vi "AOL Z Cal-Cancel handler.vi"() -> (3 "Stop?":bool)   [LabVIEW 2020]
uses:
  Globals/gl_Calibration globals.vi
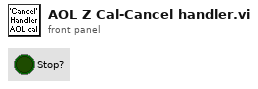
[diagram p1: front panel]
types:
  T1 = typedef "AOL Z cal process refs.ctl" = cluster{"This VI":refnum<vi>, "Abort (ind)":refnum<vi>, "Next (ind)":refnum<vi>, "Cancel":refnum<vi>, "Next":refnum<vi>, "Message":refnum<vi>, "Progress":refnum<vi>}
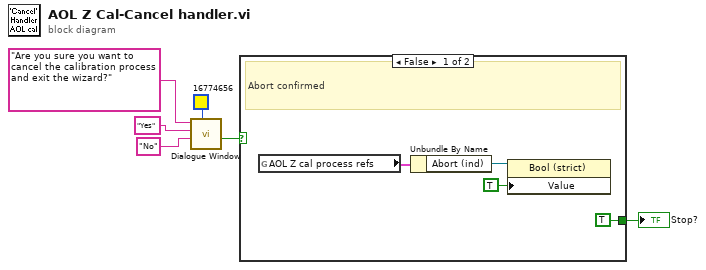
[diagram p0: block diagram]
diagram:
  n1 = call "Dialogue Window.vi"("Colour"=u32 16774656, "Caption-Left button (Cancel)"="No", "Caption-Right button (OK)"="Yes", "Message string"="Are you sure you want to cancel the calibration process and exit the wizard?") -> ("Cancelled (Left button pressed)"=w5:bool)  [unwired: 5 in, 2 out]
  n2 = case shown="False" w5 {
    tunnel: [TRUE ("Stop?") _] -> w6
    frame False {
      # "Abort confirmed"
      n3 = global read "gl_Calibration globals.vi" "AOL Z cal process refs"() -> (w8:T1)
      n4 = Unbundle By Name(w8) -> ("Abort (ind)"=w7:refnum<vi>)
      n5 = property class="Bool (strict)"(reference=w7, "Value"=TRUE) -> ()  [unwired: 1 in, 2 out]
    }
    frame True {
      # "Abort was cancelled..\nSo continue"
    }
  }
  "Stop?" <- w6
